vi "CAPTH-Find Start Condition.vi"(0 "nominal start atten":dbl, 5 "Response in":T1={"Averages (3dB steps)"=12, "Time Window (ms)"=8.5, "dt (us)"=10.0, "Grass gain"=1000.0, "CRITERION (mV)"=5.0, "CEILING (dB atten)"=20.0, "Use previous"=FALSE, "Save avgs"=FALSE, "Save raw"=FALSE, "Save history"=FALSE, "CEILING (dB SPL)"=6.0} {"CRITERION (mV)" format="%.2f"; "Time Window (ms)" format="%.2f"}, 7 "ear":i32, 9 "freq":i32, 12 "last data":T3(array[cluster]), 13 "data":T4(array[cluster])) -> (4 "start atten":dbl, 6 "Max SPL":dbl, 8 "Response out":T1={"Averages (3dB steps)"=12, "Time Window (ms)"=8.5, "dt (us)"=10.0, "Grass gain"=1000.0, "CRITERION (mV)"=60.0, "CEILING (dB atten)"=6.0, "Use previous"=FALSE, "Save avgs"=FALSE, "Save raw"=FALSE, "Save history"=FALSE, "CEILING (dB SPL)"=6.0} {"CRITERION (mV)" format="%.2f"; "Time Window (ms)" format="%.2f"}, 10 "stimcon":T2)   [LabVIEW 2020]
uses:
  Typedefs/CAPTH-Response.ctl
  Typedefs/CAPTH-StimCon.ctl
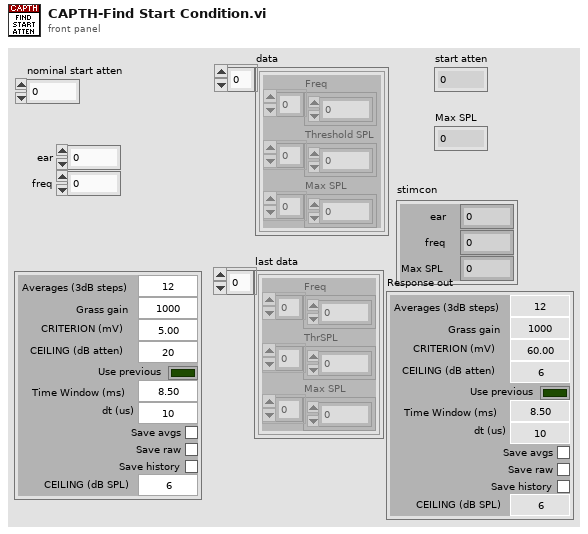
[diagram p1: front panel]
types:
  T1 = typedef "CAPTH-Response.ctl" = cluster{"Averages (3dB steps)":i32, "Time Window (ms)":dbl, "dt (us)":dbl, "Grass gain":dbl, "CRITERION (mV)":dbl, "CEILING (dB atten)":dbl, "Use previous":bool, "Save avgs":bool, "Save raw":bool, "Save history":bool, "CEILING (dB SPL)":dbl}
  T2 = typedef "CAPTH-StimCon.ctl" = cluster{"ear":i32, "freq":i32, "Max SPL":dbl}
  T3 = cluster{"Freq":dbl[], "ThrSPL":dbl[], "Max SPL":dbl[]}[]
  T4 = cluster{"Freq":dbl[], "Threshold SPL":dbl[], "Max SPL":dbl[]}[]
  T5 = cluster{"Freq":dbl[], "Threshold SPL":dbl[], "Max SPL":dbl[]}
  T6 = cluster{"Freq":dbl[], "ThrSPL":dbl[], "Max SPL":dbl[]}
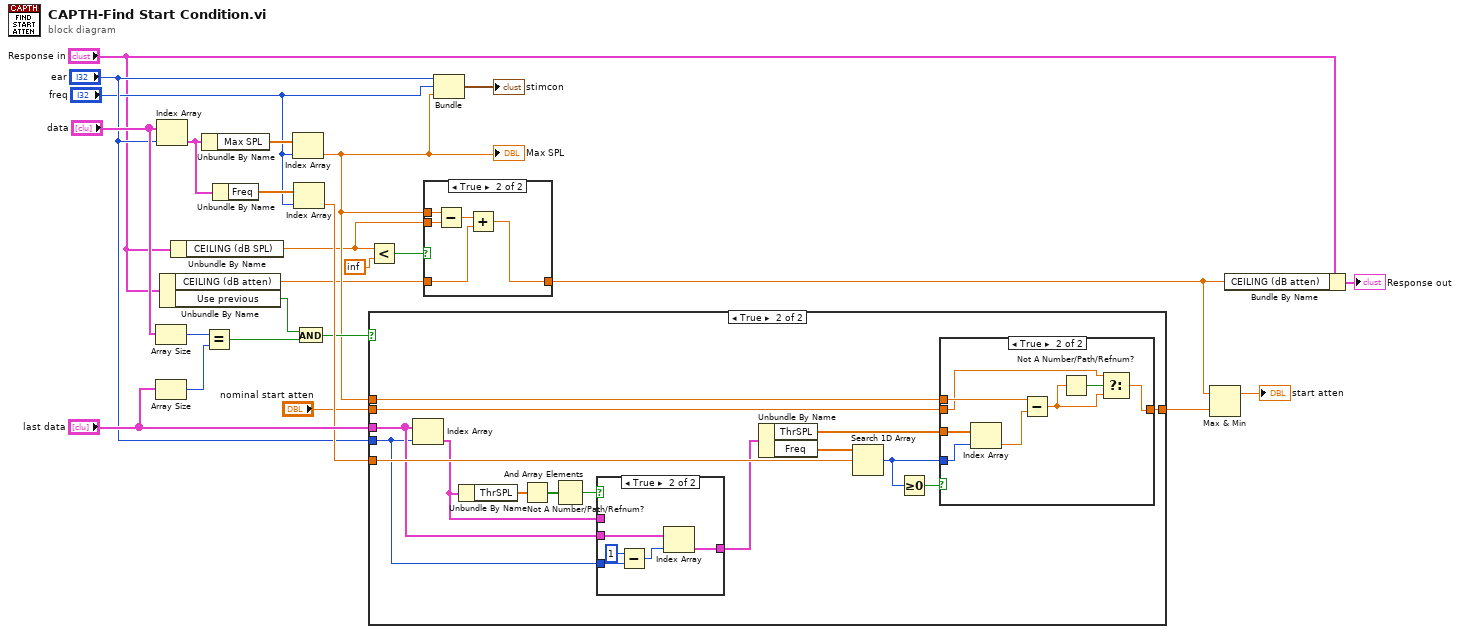
[diagram p0: block diagram]
diagram:
  n1 = Array Size(array="data") -> (size(s)=w23:i32)
  n2 = Array Size(array="last data") -> (size(s)=w22:i32)
  n3 = Index Array(array="data", index="ear") -> (element=w18:T5)
  n4 = Unbundle By Name("Response in") -> ("CEILING (dB atten)"=w5:dbl, "Use previous"=w14:bool)
  n5 = Unbundle By Name("Response in") -> ("CEILING (dB SPL)"=w7:dbl)
  n6 = Unbundle By Name(w18) -> ("Max SPL"=w25:dbl[])
  n7 = Equal?(x=w23, y=w22) -> (x = y?=w21:bool)
  n8 = Unbundle By Name(w18) -> ("Freq"=w19:dbl[])
  n9 = Index Array(array=w25, index="freq") -> (element=w9:dbl)
  "Max SPL" <- w9
  n10 = Index Array(array=w19, index="freq") -> (element=w17:dbl)
  n11 = And(x=w14, y=w21) -> (x .and. y?=w15:bool)
  n12 = Less?(x=w7, y=inf) -> (x < y?=w4:bool)
  n13 = case shown="True" w15 {
    tunnel: "last data" -> [_ w28]
    tunnel: "ear" -> [_ w27]
    tunnel: w17 -> [_ w40]
    tunnel: w9 -> [_ w37]
    tunnel: [w26 w36] -> w13
    tunnel: "nominal start atten" -> [w26 w35]
    frame False {
    }
    frame True {
      n14 = Index Array(array=w28, index=w27) -> (element=w30:T6)
      n15 = Unbundle By Name(w30) -> ("ThrSPL"=w32:dbl[])
      n16 = Not A Number/Path/Refnum?(number/path/refnum=w32) -> (NaN/Path/Refnum?=w33:bool[])
      n17 = And Array Elements(Boolean array=w33) -> (logical AND=w31:bool)
      n18 = case shown="True" w31 {
        tunnel: [w42 w46] -> w29
        tunnel: w30 -> [w42 _]
        tunnel: w28 -> [_ w47]
        tunnel: w27 -> [_ w45]
        frame False {
        }
        frame True {
          n19 = Subtract(x=1, y=w45) -> (x-y=w43:i32)
          n20 = Index Array(array=w47, index=w43) -> (element=w46:T6)
        }
      }
      n21 = Unbundle By Name(w29) -> ("ThrSPL"=w34:dbl[], "Freq"=w41:dbl[])
      n22 = Search 1D Array(1D array=w41, element=w40) -> (index of element=w38:i32)  [unwired: 1 in]
      n23 = Greater Or Equal To 0?(x=w38) -> (x >= 0?=w39:bool)
      n24 = case shown="True" w39 {
        tunnel: w38 -> [_ w55]
        tunnel: w34 -> [_ w56]
        tunnel: w37 -> [_ w54]
        tunnel: [w48 w49] -> w36
        tunnel: w35 -> [w48 w50]
        frame False {
        }
        frame True {
          n25 = Index Array(array=w56, index=w55) -> (element=w53:dbl)
          n26 = Subtract(x=w54, y=w53) -> (x-y=w51:dbl)
          n27 = Not A Number/Path/Refnum?(number/path/refnum=w51) -> (NaN/Path/Refnum?=w52:bool)
          n28 = Select(t=w50, s=w52, f=w51) -> (s? t:f=w49:dbl)
        }
      }
    }
  }
  n29 = case shown="True" w4 {
    tunnel: w9 -> [_ w62]
    tunnel: w7 -> [_ w61]
    tunnel: w5 -> [w57 w59]
    tunnel: [w57 w58] -> w2
    frame False {
    }
    frame True {
      n30 = Subtract(x=w62, y=w61) -> (x-y=w60:dbl)
      n31 = Add(x=w60, y=w59) -> (x+y=w58:dbl)
    }
  }
  n32 = Bundle("ear"="ear", "freq"="freq", w9) -> (→"stimcon":cluster{"ear":i32, "freq":i32, dbl})  [unwired: 1 in]
  n33 = Max & Min(x=w2, y=w13) -> (max(x,y)=→"start atten":dbl)  [unwired: 1 out]
  n34 = Bundle By Name(cluster="Response in", "CEILING (dB atten)"=w2) -> (→"Response out":T1)
